vi "clients_global.vi"() -> ()   [LabVIEW 2024]
panel:
  in  "Cluster":T1
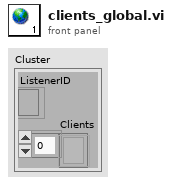
[diagram p1: front panel]
types:
  T1 = cluster{"ListenerID":refnum<k5>, "Clients":refnum<k5>[]}
diagram:
